vi "2019-05-08_01.vi"() -> ()   [LabVIEW 2018]
panel:
  out "Min Index":dbl
  out "Min":dbl
  out "Max Index":dbl
  out "Max":dbl
  out "Threshold index":dbl
  out "Match Index":dbl
  out "Element":dbl
  in  "인덱스":dbl
  out "Array Size":dbl
  in  "Numeric":dbl
  out "Array Subset":dbl[](array[numeric])
  out "Initialize Array":dbl[](array[numeric])
  out "Insert Array":dbl[](array[numeric])
  out "Reverse Array":dbl[](array[numeric])
  out "Sort Array":dbl[](array[numeric])
  out "Ratate Array":dbl[](array[numeric])
  out "Build Array":dbl[](array[numeric])
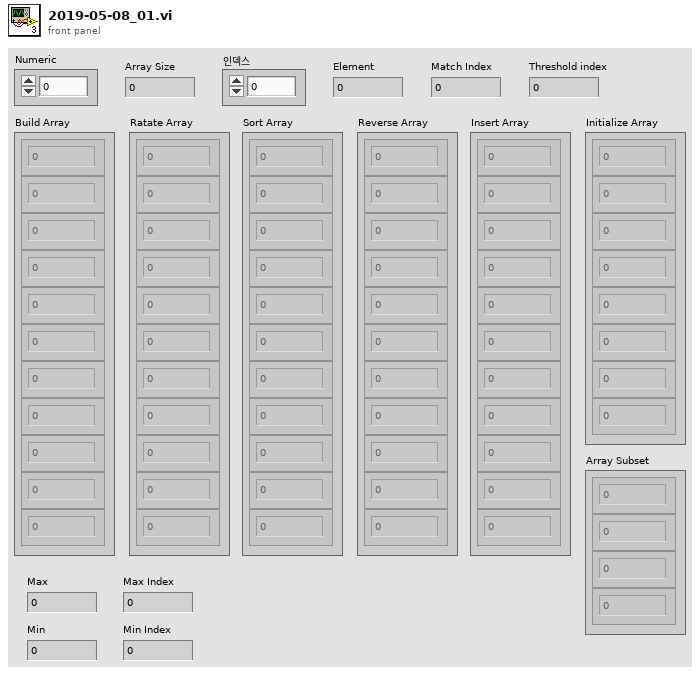
[diagram p1: front panel]
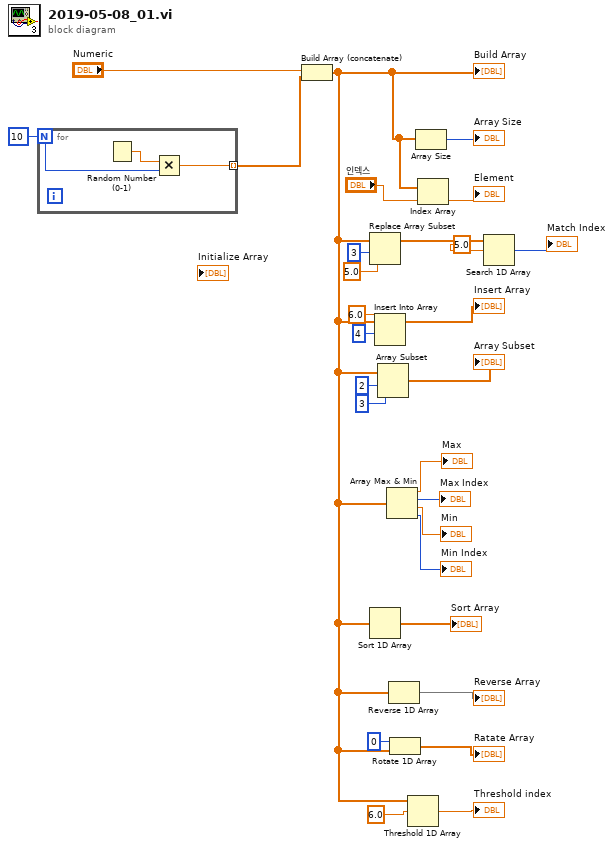
[diagram p0: block diagram]
diagram:
  n1 = for {
    N: 10 -> [w31]
    tunnel: [w29] -> w26 mode=indexing
    n2 = Random Number (0-1)() -> (number: 0 to 1=w30:dbl)
    n3 = Multiply(x=w30, y=w31) -> (x*y=w29:dbl)
  }
  n4 = Build Array (concatenate)("Numeric", w26) -> (w3:dbl[])
  "Build Array" <- w3
  n5 = Replace Array Subset(array=w3, new element=5.0 ("새 원소/부분배열"), index=3 ("인덱스")) -> (w18:dbl[])
  n6 = Sort 1D Array(array=w3) -> (sorted array=→"Sort Array":dbl[])
  n7 = Insert Into Array(array=w3, index=4 ("인덱스"), new element=6.0 ("새 원소/부분배열")) -> (→"Insert Array":dbl[])
  n8 = Array Subset(array=w3, index=2 ("인덱스"), length=3 ("길이")) -> (→"Array Subset":dbl[])
  n9 = Array Max & Min(array=w3) -> (max value=→"Max":dbl, max index (indices)=→"Max Index":i32, min value=→"Min":dbl, min index (indices)=→"Min Index":i32)
  n10 = Reverse 1D Array(array=w3) -> (reversed array=→"Reverse Array":dbl[])
  n11 = Rotate 1D Array(1:w3, 2:0 ("n")) -> (0:→"Ratate Array":dbl[])
  n12 = Threshold 1D Array(2:6.0 ("소수 인덱스 또는 x"), 3:w3) -> (0:→"Threshold index":dbl)  [unwired: 1 in]
  n13 = Array Size(array=w3) -> (size(s)=→"Array Size":i32)
  n14 = Index Array(array=w3, index="인덱스") -> (element=→"Element":dbl)
  n15 = Search 1D Array(1D array=w18, element=5.0 ("원소")) -> (index of element=→"Match Index":i32)  [unwired: 1 in]
